vi "Velocity_Enemy_Robots.vi"(9 "Pick_ID":i32, 11 "enemy_robots":T1[](array[typedef])) -> (3 "Vel_Enemy_Robots":dbl(graph))   [LabVIEW 2016]
uses:
  Core/AI Robot.ctl
  Intel/Functions Enum.ctl
  Intel/AttackerStates.ctl
  <vilib>/Analysis/_algsub.llb/Real Vector Norm.vi
  <vilib>/Analysis/NI_AALPro.lvlib
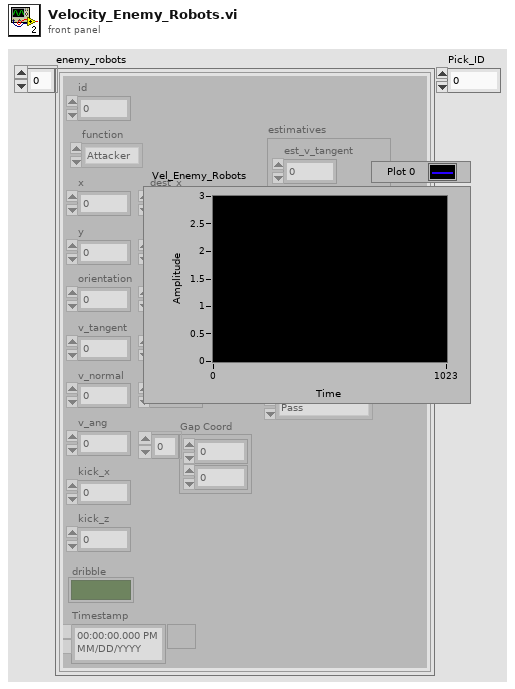
[diagram p1: front panel]
types:
  T1 = typedef "AI Robot.ctl" = cluster{"id":u32, "function":T2, "x":dbl, "y":dbl, "orientation":dbl, "v_tangent":dbl, "v_normal":dbl, "v_ang":dbl, "kick_x":dbl, "kick_z":dbl, "dribble":bool, "Timestamp":timestamp, "dest_x":dbl, "dest_y":dbl, "dest_orientation":dbl, "estimatives":cluster{"est_v_tangent":dbl, "est_v_normal":dbl, "est_vx":dbl, "est_vy":dbl, "Pos Robot Est":dbl[]}, "dest_x_kick":dbl, "dest_y_kick":dbl, "Gap Coord":dbl[], "States":T3}
  T2 = typedef "Functions Enum.ctl" = enum16{"Attacker", "Goalie", "Defender", "Striker", "Goto 0", "Dummy", "Kicker", "ZigZag"}
  T3 = typedef "AttackerStates.ctl" = enum16{"Pass", "GoToTangent", "BallGetting", "GoToKick", ""}
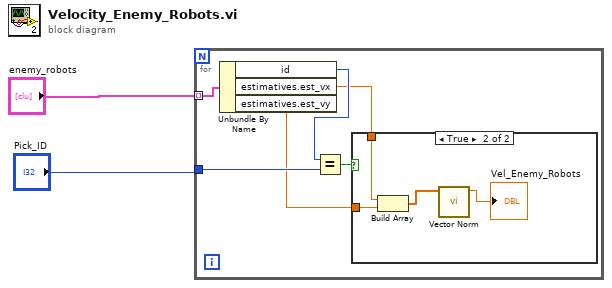
[diagram p0: block diagram]
diagram:
  n1 = for {
    tunnel: "enemy_robots" -> [w8] mode=indexing
    tunnel: "Pick_ID" -> [w6]
    n2 = Unbundle By Name(w8) -> ("id"=w5:u32, "estimatives.est_vx"=w4:dbl, "estimatives.est_vy"=w3:dbl)
    n3 = Equal?(x=w5, y=w6) -> (x = y?=w7:bool)
    n4 = case shown="True" w7 {
      tunnel: w4 -> [_ w11]
      tunnel: w3 -> [_ w10]
      frame False {
      }
      frame True {
        n5 = Build Array(w11, w10) -> (w9:dbl[])
        n6 = call-poly <vilib>:"Vector Norm.vi"("Input Vector"=w9) -> ("norm"=→"Vel_Enemy_Robots":dbl)  [unwired: 9 in, 1 out]
      }
    }
  }
